vi "RubikDoMove.vi"(0 "Value":T1) -> ()   [LabVIEW 2017]
uses:
  Projekt-RubikLibrary/RubikMoves.ctl
  Projekt-RubikLibrary/ServoEnumControl.ctl
  Projekt-RubikLibrary/ServoCCWControl.ctl
  Projekt-RubikLibrary/RubikLibrary.lvlib
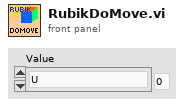
[diagram p1: front panel]
types:
  T1 = typedef "RubikLibrary.lvlib/RubikMoves.ctl" = enum16{"U", "U'", "F", "F'", "D", "D'", "B", "B'", "L", "L'", "R", "R'"}
  T2 = typedef "RubikLibrary.lvlib/ServoCCWControl.ctl" = enum16{"cw", "ccw"}
  T3 = typedef "RubikLibrary.lvlib/ServoEnumControl.ctl" = enum16{"Left Servo", "Front Servo", "Right Servo"}
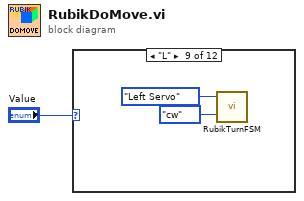
[diagram p0: block diagram]
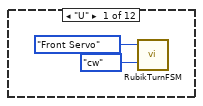
[diagram p2: hidden frame]
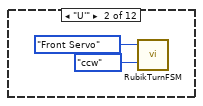
[diagram p3: hidden frame]
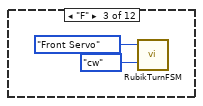
[diagram p4: hidden frame]
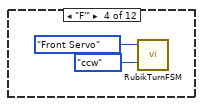
[diagram p5: hidden frame]
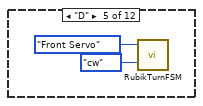
[diagram p6: hidden frame]
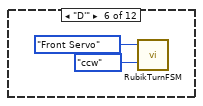
[diagram p7: hidden frame]
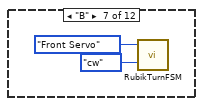
[diagram p8: hidden frame]
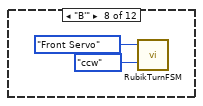
[diagram p9: hidden frame]
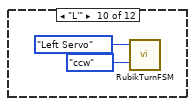
[diagram p10: hidden frame]
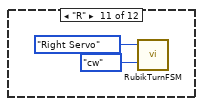
[diagram p11: hidden frame]
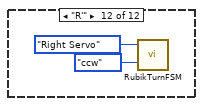
[diagram p12: hidden frame]
diagram:
  n1 = case shown="\"L\"" "Value" {
    frame "U" {
      n2 = call "RubikTurnFSM.vi"("Turn"=ServoCCWControl."cw", "Servo"=ServoEnumControl."Front Servo") -> ()  [unwired: 2 in, 2 out]
    }
    frame "U'" {
      n3 = call "RubikTurnFSM.vi"("Turn"=ServoCCWControl."ccw", "Servo"=ServoEnumControl."Front Servo") -> ()  [unwired: 2 in, 2 out]
    }
    frame "F" {
      n4 = call "RubikTurnFSM.vi"("Turn"=ServoCCWControl."cw", "Servo"=ServoEnumControl."Front Servo") -> ()  [unwired: 2 in, 2 out]
    }
    frame "F'" {
      n5 = call "RubikTurnFSM.vi"("Turn"=ServoCCWControl."ccw", "Servo"=ServoEnumControl."Front Servo") -> ()  [unwired: 2 in, 2 out]
    }
    frame "D" {
      n6 = call "RubikTurnFSM.vi"("Turn"=ServoCCWControl."cw", "Servo"=ServoEnumControl."Front Servo") -> ()  [unwired: 2 in, 2 out]
    }
    frame "D'" {
      n7 = call "RubikTurnFSM.vi"("Turn"=ServoCCWControl."ccw", "Servo"=ServoEnumControl."Front Servo") -> ()  [unwired: 2 in, 2 out]
    }
    frame "B" {
      n8 = call "RubikTurnFSM.vi"("Turn"=ServoCCWControl."cw", "Servo"=ServoEnumControl."Front Servo") -> ()  [unwired: 2 in, 2 out]
    }
    frame "B'" {
      n9 = call "RubikTurnFSM.vi"("Turn"=ServoCCWControl."ccw", "Servo"=ServoEnumControl."Front Servo") -> ()  [unwired: 2 in, 2 out]
    }
    frame "L" {
      n10 = call "RubikTurnFSM.vi"("Turn"=ServoCCWControl."cw", "Servo"=ServoEnumControl."Left Servo") -> ()  [unwired: 2 in, 2 out]
    }
    frame "L'" {
      n11 = call "RubikTurnFSM.vi"("Turn"=ServoCCWControl."ccw", "Servo"=ServoEnumControl."Left Servo") -> ()  [unwired: 2 in, 2 out]
    }
    frame "R" {
      n12 = call "RubikTurnFSM.vi"("Turn"=ServoCCWControl."cw", "Servo"=ServoEnumControl."Right Servo") -> ()  [unwired: 2 in, 2 out]
    }
    frame "R'" {
      n13 = call "RubikTurnFSM.vi"("Turn"=ServoCCWControl."ccw", "Servo"=ServoEnumControl."Right Servo") -> ()  [unwired: 2 in, 2 out]
    }
  }
